vi "Disconnect.vi"(8 "error in":errorcluster, 11 "2936r in":refnum<class "2936r.lvclass">) -> (0 "error out":errorcluster, 3 "2936r out":refnum<class "2936r.lvclass">)   [LabVIEW 2018, in "2936r.lvlib" / "2936r.lvclass"]
uses:
  2936r.lvclass
  2936r.lvclass/2936r.ctl
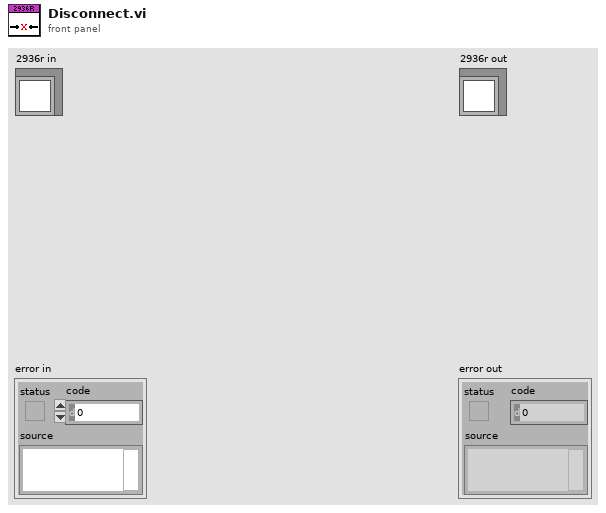
[diagram p1: front panel]
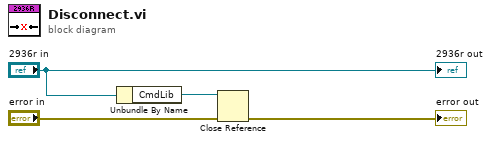
[diagram p0: block diagram]
diagram:
  n1 = Unbundle By Name("2936r in") -> ("CmdLib"=w4:refnum<k24>)
  n2 = Close Reference(reference=w4, error in (no error)="error in") -> (error out=→"error out":errorcluster)
  "2936r out" <- "2936r in"
